vi "insert_bytes.vi"(9 "offset (-1: current position)":i32=-1, 10 "bytes to insert":refnum<class "Bytes.lvclass">, 11 "Bytes in":refnum<class "Bytes.lvclass">) -> (3 "Bytes out":refnum<class "Bytes.lvclass">)   [LabVIEW 2020, in "variant.lvlib" / "Bytes.lvclass"]
uses:
  Bytes.lvclass
  Bytes.lvclass/Bytes.ctl
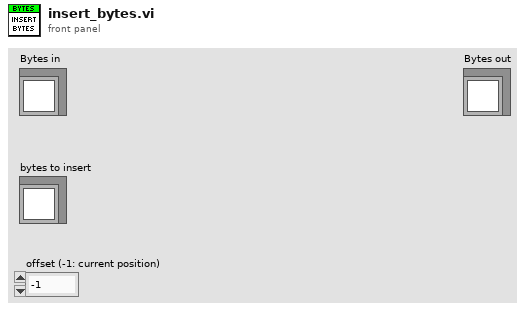
[diagram p1: front panel]
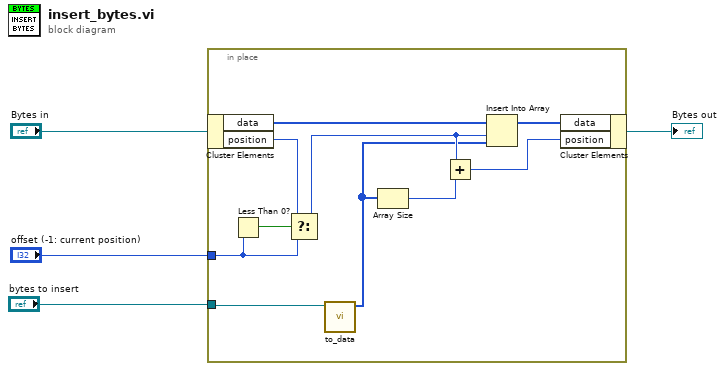
[diagram p0: block diagram]
diagram:
  n1 = in-place {
    in-place-border: "offset (-1: current position)" -> [w12]
    in-place-border: "bytes to insert" -> [w11]
    n2 = in-place-cluster #1("Bytes in") -> ("data"=w8:u8[], "position"=w13:i32)
    n3 = Less Than 0?(x=w12) -> (x < 0?=w14:bool)
    n4 = Select(t=w13, s=w14, f=w12) -> (s? t:f=w6:i32)
    n5 = call "to_data.vi"("Bytes in"=w11) -> ("byte array"=w5:u8[])  [unwired: 10 in]
    n6 = Array Size(array=w5) -> (size(s)=w10:i32)
    n7 = Add(x=w6, y=w10) -> (x+y=w9:i32)
    n8 = Insert Into Array(array=w8, index=w6, new element=w5) -> (w7:u8[])
    n9 = in-place-cluster #1("data"=w7, "position"=w9) -> (→"Bytes out":refnum<class "Bytes.lvclass">)
  }
